vi "Read Water Level Actor.vi"(11 "蒸发冷却器":refnum<class "Evaporative Cooler.lvclass">) -> (2 "水位":refnum<class "Water Level.lvclass">)   [LabVIEW 2013, in "Evaporative Cooler.lvlib" / "Evaporative Cooler.lvclass"]
doc: "读取“水位”操作者，该操作者应由蒸发冷却器负责启动。子类中必须对该方法进行重写以返回符合应用需要的水位。例如，仿真的蒸发冷却器需要返回仿真的水位。"
uses:
  Evaporative Cooler.lvclass
  Water Level/Water Level.lvclass
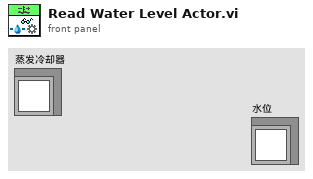
[diagram p1: front panel]
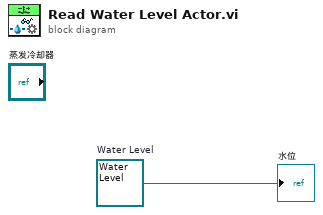
[diagram p0: block diagram]
diagram:
  w1 = refnum<class "Water Level.lvclass"> refnum  # Water Level
  "水位" <- w1
